vi "set_port.vi"(8 "error in (no error)":errorcluster, 10 "VISA resource name":refnum<visa-resource-name>, 11 "DC_power_supply in":refnum<class "DC_power_supply.lvclass">) -> (0 "error out":errorcluster, 3 "DC_power_supply out":refnum<class "DC_power_supply.lvclass">)   [LabVIEW 2017, in "DC_power_supply.lvclass"]
uses:
  DC_power_supply.lvclass
  DC_power_supply.lvclass/DC_power_supply.ctl
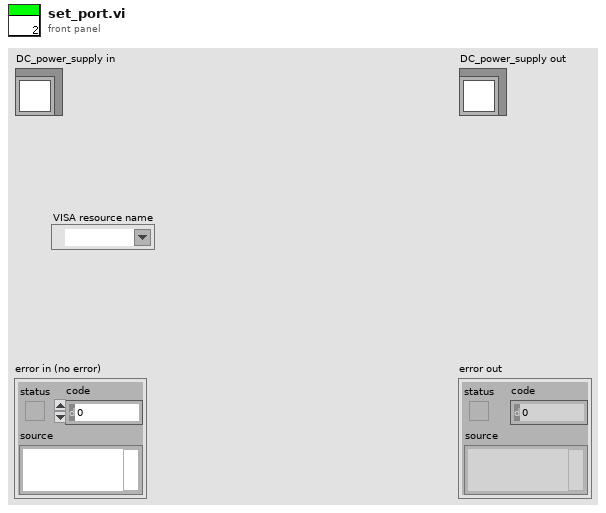
[diagram p1: front panel]
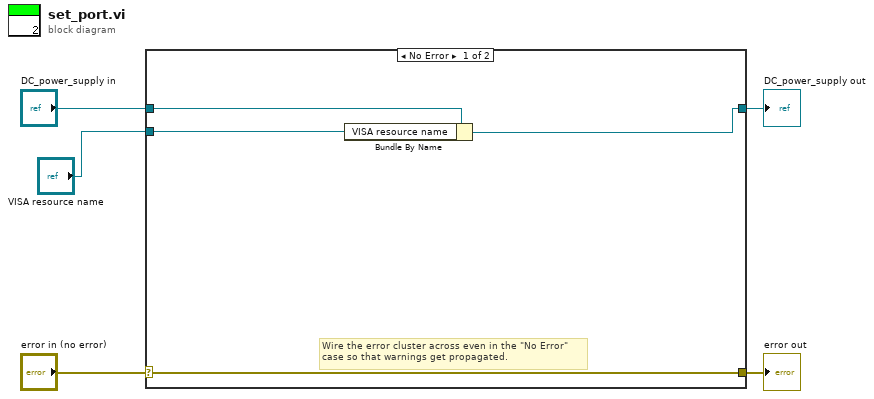
[diagram p0: block diagram]
diagram:
  n1 = case shown="No Error" "error in (no error)" {
    selector: "error in (no error)" -> [w9 w11]
    tunnel: [w9 w11] -> w4
    tunnel: [w7 w10] -> w2
    tunnel: "DC_power_supply in" -> [w8 w10]
    tunnel: "VISA resource name" -> [w6 _]
    frame No Error {
      # "Wire the error cluster across even in the \"No Error\"\ncase so that warnings get propagated."
      n2 = Bundle By Name(cluster=w8, "VISA resource name"=w6) -> (w7:refnum<class "DC_power_supply.lvclass">)
    }
    frame Error {
    }
  }
  "error out" <- w4
  "DC_power_supply out" <- w2
